vi "GenerateBrowerComponent.vi"(6 "SymbolIndex(0)":i32, 8 "error in (no error)":errorcluster, 9 "ComponentName(\"\")":string, 10 "ComponentID(\"\")":string, 11 "Factory in":refnum<class "Factory.lvclass">) -> (0 "error out":errorcluster, 2 "BrowerComponent":refnum<class "BrowerComponent.lvclass">, 3 "Factory out":refnum<class "Factory.lvclass">)   [LabVIEW 2015, in "Factory.lvclass"]
uses:
  Factory.lvclass
  BrowerComponent/BrowerComponent/BrowerComponent.lvclass
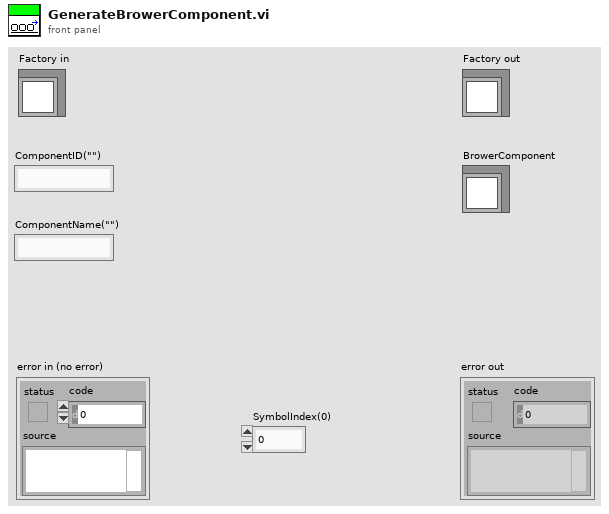
[diagram p1: front panel]
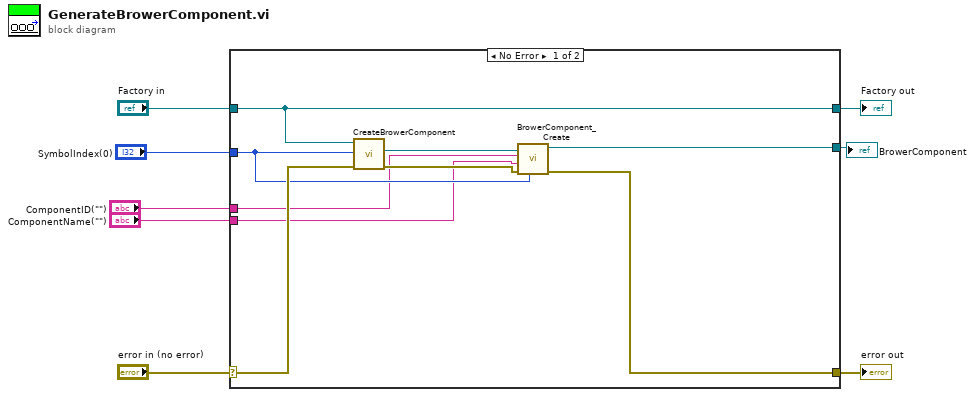
[diagram p0: block diagram]
diagram:
  n1 = case shown="No Error" "error in (no error)" {
    selector: "error in (no error)" -> [w16 w19]
    tunnel: [w13 w19] -> w7
    tunnel: [w17 w18] -> w5
    tunnel: "Factory in" -> [w17 w18]
    tunnel: "SymbolIndex(0)" -> [w12 _]
    tunnel: [w11 _] -> w3
    tunnel: "ComponentID(\"\")" -> [w10 _]
    tunnel: "ComponentName(\"\")" -> [w9 _]
    frame No Error {
      n2 = call-dynamic "CreateBrowerComponent.vi"("error in (no error)"=w16, "SymbolIndex"=w12, "BrowerFactory in"=w17) -> ("error out"=w14:errorcluster, "BrowerComponent"=w15:refnum<class "BrowerComponent.lvclass">)  [unwired: 6 in, 1 out]
      n3 = call "BrowerComponent_Create.vi"("SymbolIndex"=w12, "error in (no error)"=w14, "ComponentName"=w9, "ComponentID"=w10, "reference in"=w15) -> ("error out"=w13:errorcluster, "reference out"=w11:refnum<class "BrowerComponent.lvclass">)  [unwired: 5 in]
    }
    frame Error {
    }
  }
  "error out" <- w7
  "Factory out" <- w5
  "BrowerComponent" <- w3
